vi "流量计全局变量.vi"() -> ()   [LabVIEW 2022 SP3, in "流量计集成.lvlib"]
uses:
  <vilib>/Plasmionique/MB Master/MB_Master_Serial/MB_Master_Serial.lvclass
panel:
  in  "数量 10":u16
  in  "流量计启用 10":bool
  in  "数量 9":u16
  in  "数量 8":u16
  in  "流量计启用 9":bool
  in  "数据存储间隔(min)":u16=5
  in  "屏蔽负值":bool=TRUE
  in  "流量计启用 8":bool
  in  "数量 7":u16
  in  "流量计启用 7":bool
  in  "每小时总流量/总累积流量":bool
  out "初始化":bool
  out "MB_Serial session":refnum<class "MB_Master_Serial.lvclass">
  in  "serial port":refnum<visa-resource-name>="COM10" caption="串口"
  in  "baud rate":u32(ring)=9600 caption="波特率" items=["1200"=1200, "2400"=2400, "4800"=4800, "9600"=9600, "19200"=19200, "38400"=38400, "115200"=115200]
  in  "数量 6":u16
  in  "流量计启用 6":bool
  in  "运行模式设置":enum16{"按周期模式", "全常规模式"}(ring)=enum."全常规模式"
  in  "运行模式":enum16{"维护模式", "常规模式", "应急模式", "质控模式", "性能测试"}(ring)=enum."常规模式"
  in  "数量 5":u16
  in  "流量计启用 5":bool
  in  "流量计类型":T1
  in  "数量 4":u16
  in  "流量计启用 4":bool
  in  "流量计启用 3":bool
  in  "流量计启用 2":bool
  in  "流量计启用":bool
  in  "博意达流量计启用":bool[](array[boolean])
  in  "运行间隔":i16=4 min=1 max=24
  in  "数量 3":u16
  in  "数量 2":u16
  in  "数量":u16
  out "总累积流量":dbl
  out "总流量":dbl
  out "平均流速":dbl
  out "平均水位":dbl
  out "TX Timestamp":timestamp
  out "TX Data":string
  out "RX Timestamp":timestamp
  out "RX Data":string
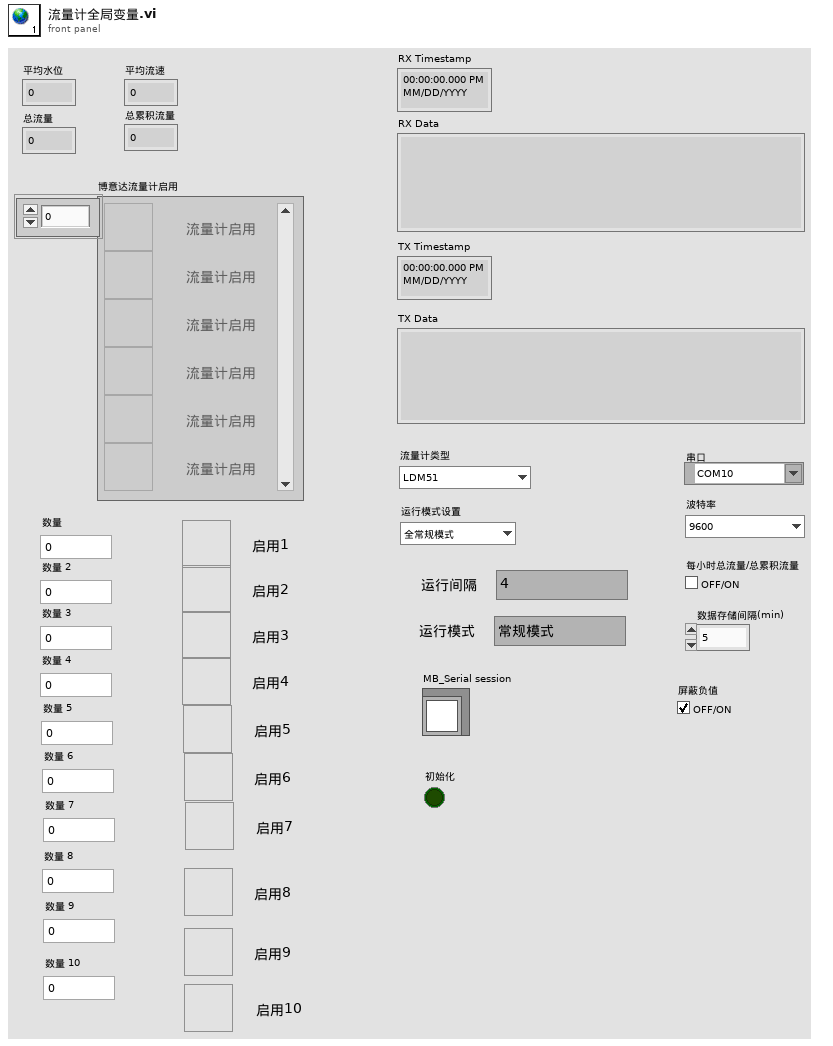
[diagram p1: front panel]
types:
  T1 = typedef "流量计集成.lvlib/流量计类型.ctl" = enum16{"LDM51", "MGG/KL QC", "斯坦道功率测流", "LSH10-1QC流量计", "SL1500-3G", "WL1A1明渠流量计", "LSS-100X流量计", "LS-H600流量计", "LS-H600 TCP Client", "压力水位计", "LSS-10Q流量计"}
diagram:
